vi "步骤簇数组.vi"(9 "簇":T1, 10 "组合框":refnum<vi>, 11 "簇 2":refnum<vi>) -> ()   [LabVIEW 2016]
panel:
  out "上次的簇":T1
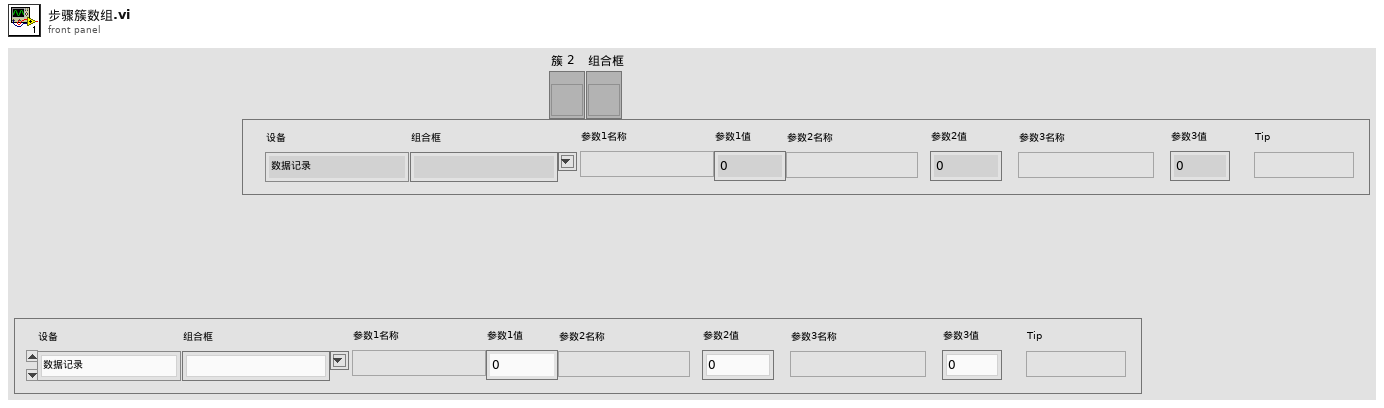
[diagram p1: front panel]
types:
  T1 = cluster{"设备":enum16{"数据记录", "Module", "VICI Valve", "其他"}, "组合框":string, "参数1名称":string, "参数1值":dbl, "参数2名称":string, "参数2值 ":dbl, "参数3名称 ":string, "参数3值  ":dbl, "Tip":string}
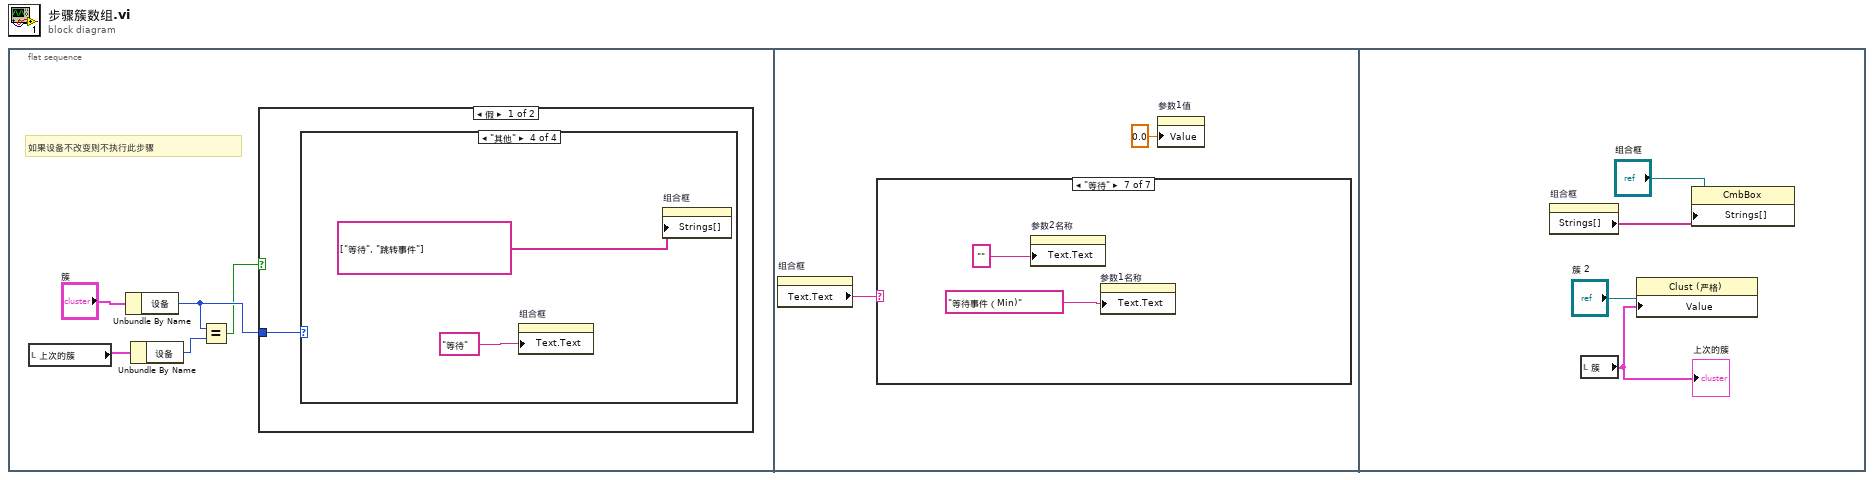
[diagram p0: block diagram]
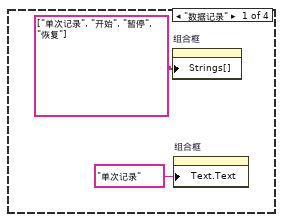
[diagram p2: hidden frame]
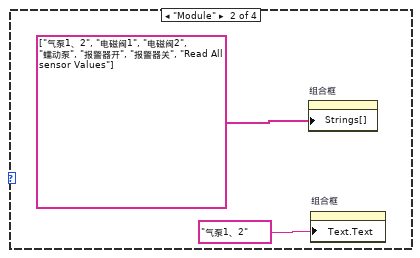
[diagram p3: hidden frame]
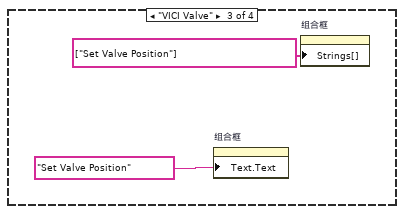
[diagram p4: hidden frame]
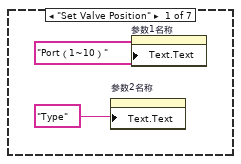
[diagram p6: hidden frame]
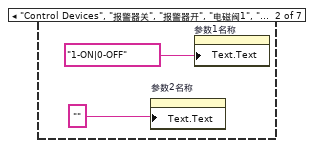
[diagram p7: hidden frame]
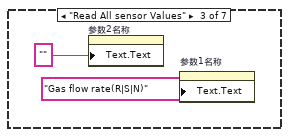
[diagram p8: hidden frame]
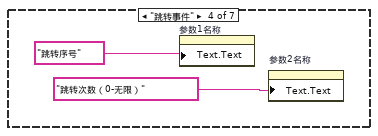
[diagram p9: hidden frame]
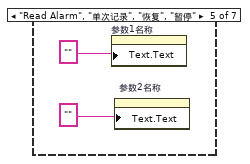
[diagram p10: hidden frame]
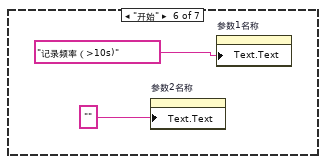
[diagram p11: hidden frame]
diagram:
  n1 = flat-sequence {
    frame #0 {
      # "如果设备不改变则不执行此步骤"
      n2 = local read "上次的簇"() -> (w4:T1)
      n3 = Unbundle By Name("簇") -> ("设备"=w3:enum16{"数据记录", "Module", "VICI Valve", "其他"})
      n4 = Unbundle By Name(w4) -> ("设备"=w2:enum16{"数据记录", "Module", "VICI Valve", "其他"})
      n5 = Equal?(x=w3, y=w2) -> (x = y?=w1:bool)
      n6 = case shown="假" w1 {
        tunnel: w3 -> [w6 _]
        frame False {
          n7 = case shown="\"其他\"" w6 {
            frame "数据记录" {
              n8 = property on="组合框" class="CmbBox"("Strings[]"=string[] ["单次记录", "开始", "暂停", "恢复"] ("字符串[]")) -> ()  [unwired: 2 in, 2 out]
              n9 = property on="组合框" class="CmbBox"("Text.Text"="单次记录" ("文本.文本")) -> ()  [unwired: 2 in, 2 out]
            }
            frame "Module" {
              n10 = property on="组合框" class="CmbBox"("Strings[]"=string[] ["气泵1、2", "电磁阀1", "电磁阀2", "蠕动泵", "报警器开", "报警器关", "Read All sensor Values"] ("字符串[]")) -> ()  [unwired: 2 in, 2 out]
              n11 = property on="组合框" class="CmbBox"("Text.Text"="气泵1、2" ("文本.文本")) -> ()  [unwired: 2 in, 2 out]
            }
            frame "VICI Valve" {
              n12 = property on="组合框" class="CmbBox"("Text.Text"="Set Valve Position" ("文本.文本")) -> ()  [unwired: 2 in, 2 out]
              n13 = property on="组合框" class="CmbBox"("Strings[]"=string[] ["Set Valve Position"] ("字符串[]")) -> ()  [unwired: 2 in, 2 out]
            }
            frame "其他" {
              n14 = property on="组合框" class="CmbBox"("Text.Text"="等待" ("文本.文本")) -> ()  [unwired: 2 in, 2 out]
              n15 = property on="组合框" class="CmbBox"("Strings[]"=string[] ["等待", "跳转事件"] ("字符串[]")) -> ()  [unwired: 2 in, 2 out]
            }
          }
        }
        frame True {
        }
      }
    }
    frame #1 {
      n16 = property on="组合框" class="CmbBox"() -> ("Text.Text"=w16:string)  [unwired: 2 in, 2 out]
      n17 = case shown="\"等待\"" w16 {
        frame "Set Valve Position" {
          n18 = property on="参数2名称" class="Str"("Text.Text"="Type" ("文本.文本")) -> ()  [unwired: 2 in, 2 out]
          n19 = property on="参数1名称" class="Str"("Text.Text"="Port（1~10）" ("文本.文本")) -> ()  [unwired: 2 in, 2 out]
        }
        frame "Control Devices", "报警器关", "报警器开", "电磁阀1", "电磁阀2", "气泵1、2", "蠕动泵", Default {
          n20 = property on="参数2名称" class="Str"("Text.Text"="" ("文本.文本")) -> ()  [unwired: 2 in, 2 out]
          n21 = property on="参数1名称" class="Str"("Text.Text"="1-ON|0-OFF" ("文本.文本")) -> ()  [unwired: 2 in, 2 out]
        }
        frame "Read All sensor Values" {
          n22 = property on="参数2名称" class="Str"("Text.Text"="" ("文本.文本")) -> ()  [unwired: 2 in, 2 out]
          n23 = property on="参数1名称" class="Str"("Text.Text"="Gas flow rate(R|S|N)" ("文本.文本")) -> ()  [unwired: 2 in, 2 out]
        }
        frame "跳转事件" {
          n24 = property on="参数1名称" class="Str"("Text.Text"="跳转序号" ("文本.文本")) -> ()  [unwired: 2 in, 2 out]
          n25 = property on="参数2名称" class="Str"("Text.Text"="跳转次数（0-无限）" ("文本.文本")) -> ()  [unwired: 2 in, 2 out]
        }
        frame "Read Alarm", "单次记录", "恢复", "暂停" {
          n26 = property on="参数1名称" class="Str"("Text.Text"="" ("文本.文本")) -> ()  [unwired: 2 in, 2 out]
          n27 = property on="参数2名称" class="Str"("Text.Text"="" ("文本.文本")) -> ()  [unwired: 2 in, 2 out]
        }
        frame "开始" {
          n28 = property on="参数2名称" class="Str"("Text.Text"="" ("文本.文本")) -> ()  [unwired: 2 in, 2 out]
          n29 = property on="参数1名称" class="Str"("Text.Text"="记录频率（>10s)" ("文本.文本")) -> ()  [unwired: 2 in, 2 out]
        }
        frame "等待" {
          n30 = property on="参数2名称" class="Str"("Text.Text"="" ("文本.文本")) -> ()  [unwired: 2 in, 2 out]
          n31 = property on="参数1名称" class="Str"("Text.Text"="等待事件（Min)" ("文本.文本")) -> ()  [unwired: 2 in, 2 out]
        }
      }
      n32 = property on="参数1值" class="DigNum (严格)"("Value"=0.0 ("值")) -> ()  [unwired: 2 in, 2 out]
    }
    frame #2 {
      n33 = property on="组合框" class="CmbBox"() -> ("Strings[]"=w31:string[])  [unwired: 2 in, 2 out]
      n34 = local read "簇"() -> (w33:T1)
      "上次的簇" <- w33
      n35 = property class="Clust (严格)"(reference="簇 2", "Value"=w33) -> ()  [unwired: 1 in, 2 out]
      n36 = property class="CmbBox"(reference="组合框", "Strings[]"=w31) -> ()  [unwired: 1 in, 2 out]
    }
  }
